vi "6-8素材.vi"() -> ()   [LabVIEW 2018]
uses:
  <vilib>/measure/maspectr.llb/FFT Spectrum (Mag-Phase) for 1 Chan.vi
  <vilib>/measure/maspectr.llb/FFT Spectrum (Mag-Phase) for N Chan.vi
  <vilib>/measure/macond.llb/IIR Filter for 1 Chan.vi
  <vilib>/measure/NI_MABase.lvlib
  <vilib>/measure/NI_MAPro.lvlib
panel:
  in  "IIR filter specifications":T1={"Topology"=enum."Butterworth", "Type"=enum."Lowpass", "Order"=1, "Lower Fc"=100.0, "Upper Fc"=200.0, "PB Ripple"=1.0, "SB Attenuation"=60.0} caption="IIR滤波器规范" {"PB Ripple" format="%0.2f"; "SB Attenuation" format="%0.2f"; "Lower Fc" format="%0.2p"; "Upper Fc" format="%0.2p"}
  in  "噪声幅值":dbl(slide) scale=0.0..1.0
  in  "选项卡控件":enum32{"调制", "滤波"}(tab)
  out "混频后频谱图":cluster{"f0":dbl, "df":dbl, "magnitude":dbl[]}(graph)
  out "两个信号频域图":cluster{"f0":dbl, "df":dbl, "magnitude":dbl[]}[](graph)
  out "混频时域图":waveform(dbl)(graph)
  out "两个信号时域图":waveform(dbl)[](graph)
  out "解调后时域":waveform(dbl)(graph)
  out "相干后时域":waveform(dbl)(graph)
  out "相干后频谱":cluster{"f0":dbl, "df":dbl, "magnitude":dbl[]}(graph)
  out "解调后频谱":cluster{"f0":dbl, "df":dbl, "magnitude":dbl[]}(graph)
  in  "调制系数":dbl(slide) min=0.0 max=1.0 scale=0.0..1.0
  in  "信号频率":dbl(slide)=10.0 min=0.0 max=10.0 scale=0.0..10.0
  in  "signal type":T2(ring) caption="信号类型"
  in  "载波频率":dbl(slide)=40.0 min=40.0 max=100.0 scale=40.0..100.0
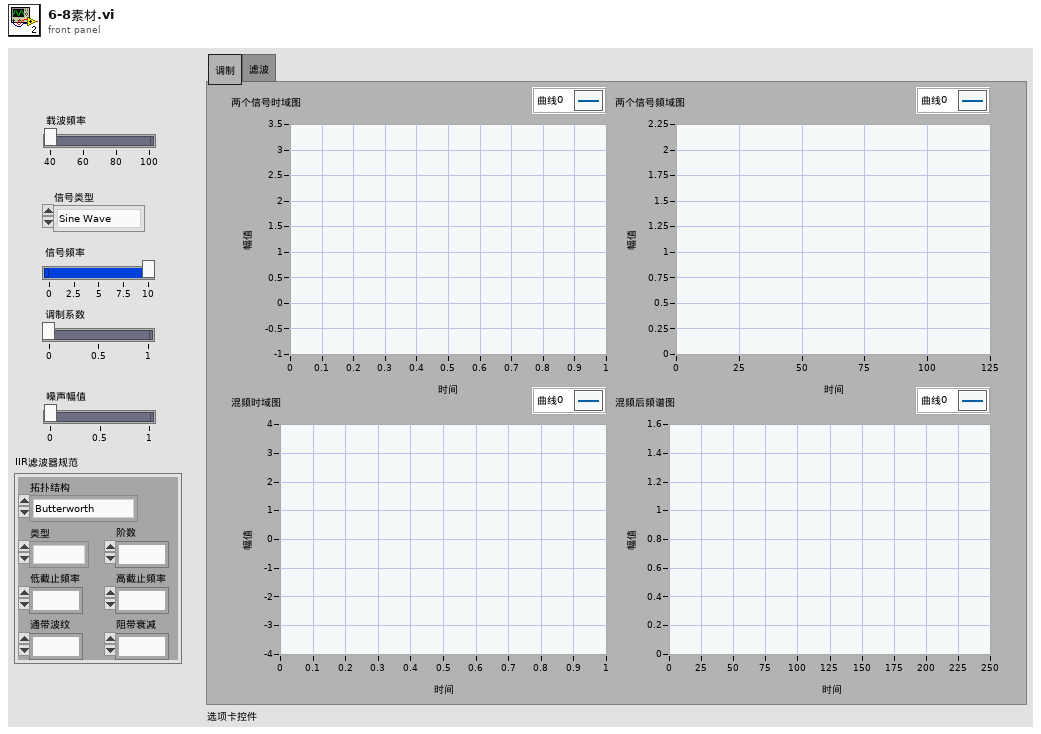
[diagram p1: front panel]
types:
  T1 = cluster{"Topology":enum16{"Off", "Butterworth", "Chebyshev", "Inverse Chebyshev", "Elliptic", "Bessel"}, "Type":enum16{"Lowpass", "Highpass", "Bandpass", "Bandstop"}, "Order":i32, "Lower Fc":dbl, "Upper Fc":dbl, "PB Ripple":dbl, "SB Attenuation":dbl}
  T2 = enum16{"Sine Wave", "Triangle Wave", "Square Wave", "Sawtooth Wave"}
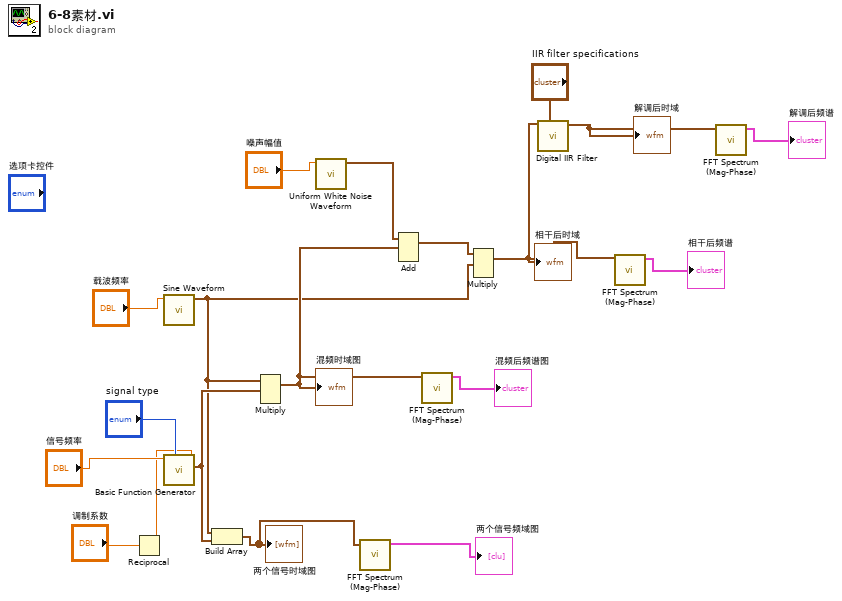
[diagram p0: block diagram]
diagram:
  n1 = Reciprocal(x="调制系数") -> (1/x=w15:dbl)
  n2 = call <vilib>:"Sine Waveform.vi"("frequency"="载波频率") -> ("signal out"=w6:waveform(dbl))  [unwired: 9 in, 1 out]
  n3 = call <vilib>:"Basic Function Generator.vi"("offset"=w15, "signal type"="signal type", "frequency"="信号频率") -> ("signal out"=w14:waveform(dbl))  [unwired: 6 in, 2 out]
  n4 = Build Array(w6, w14) -> (w13:waveform(dbl)[])
  "两个信号时域图" <- w13
  n5 = Multiply(1:w14, 2:w6) -> (0:w8:waveform(dbl))  [unwired: 1 in, 1 out]
  "混频时域图" <- w8
  n6 = call <vilib>:"Uniform White Noise Waveform.vi"("amplitude"="噪声幅值") -> ("signal out"=w9:waveform(dbl))  [unwired: 9 in, 1 out]
  n7 = call-poly <vilib>:"FFT Spectrum (Mag-Phase).vi"("time signals"=w13) -> ("magnitudes"=→"两个信号频域图":cluster{"f0":dbl, "df":dbl, "magnitude":dbl[]}[])  [unwired: 6 in, 4 out]
  n8 = Add(1:w8, 2:w9) -> (0:w7:waveform(dbl))  [unwired: 1 in, 1 out]
  n9 = call-poly <vilib>:"FFT Spectrum (Mag-Phase).vi"("time signal"=w8) -> ("magnitude"=→"混频后频谱图":cluster{"f0":dbl, "df":dbl, "magnitude":dbl[]})  [unwired: 6 in, 4 out]
  n10 = Multiply(1:w6, 2:w7) -> (0:w4:waveform(dbl))  [unwired: 1 in, 1 out]
  "相干后时域" <- w4
  n11 = call-poly <vilib>:"Digital IIR Filter.vi"("IIR filter specifications"="IIR filter specifications", "signal in"=w4) -> ("signal out"=w1:waveform(dbl))  [unwired: 7 in, 2 out]
  "解调后时域" <- w1
  n12 = call-poly <vilib>:"FFT Spectrum (Mag-Phase).vi"("time signal"=w4) -> ("magnitude"=→"相干后频谱":cluster{"f0":dbl, "df":dbl, "magnitude":dbl[]})  [unwired: 6 in, 4 out]
  n13 = call-poly <vilib>:"FFT Spectrum (Mag-Phase).vi"("time signal"=w1) -> ("magnitude"=→"解调后频谱":cluster{"f0":dbl, "df":dbl, "magnitude":dbl[]})  [unwired: 6 in, 4 out]
